vi "Mixed mode s-parameter - change port assignment.vi"(11 "S-parameters in":cdb[][](array[numeric]) format="%#.6g") -> (3 "S-parameters out":cdb[][](array[numeric]) format="%#.6g")   [LabVIEW 2020]
uses:
  <vilib>/addons/HF Network Analysis/Support VIs/Read SnP File (SnP).vi
  <vilib>/addons/HF Network Analysis/NI_HFNetworkAnalysis.lvlib
panel:
  in  "Run Standalone":bool
  in  "SnP File Path":path
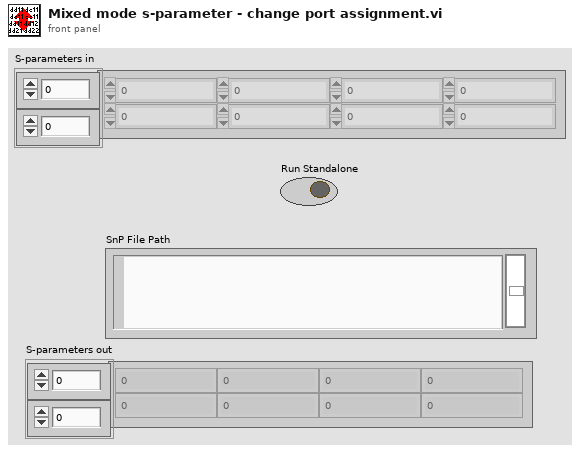
[diagram p1: front panel]
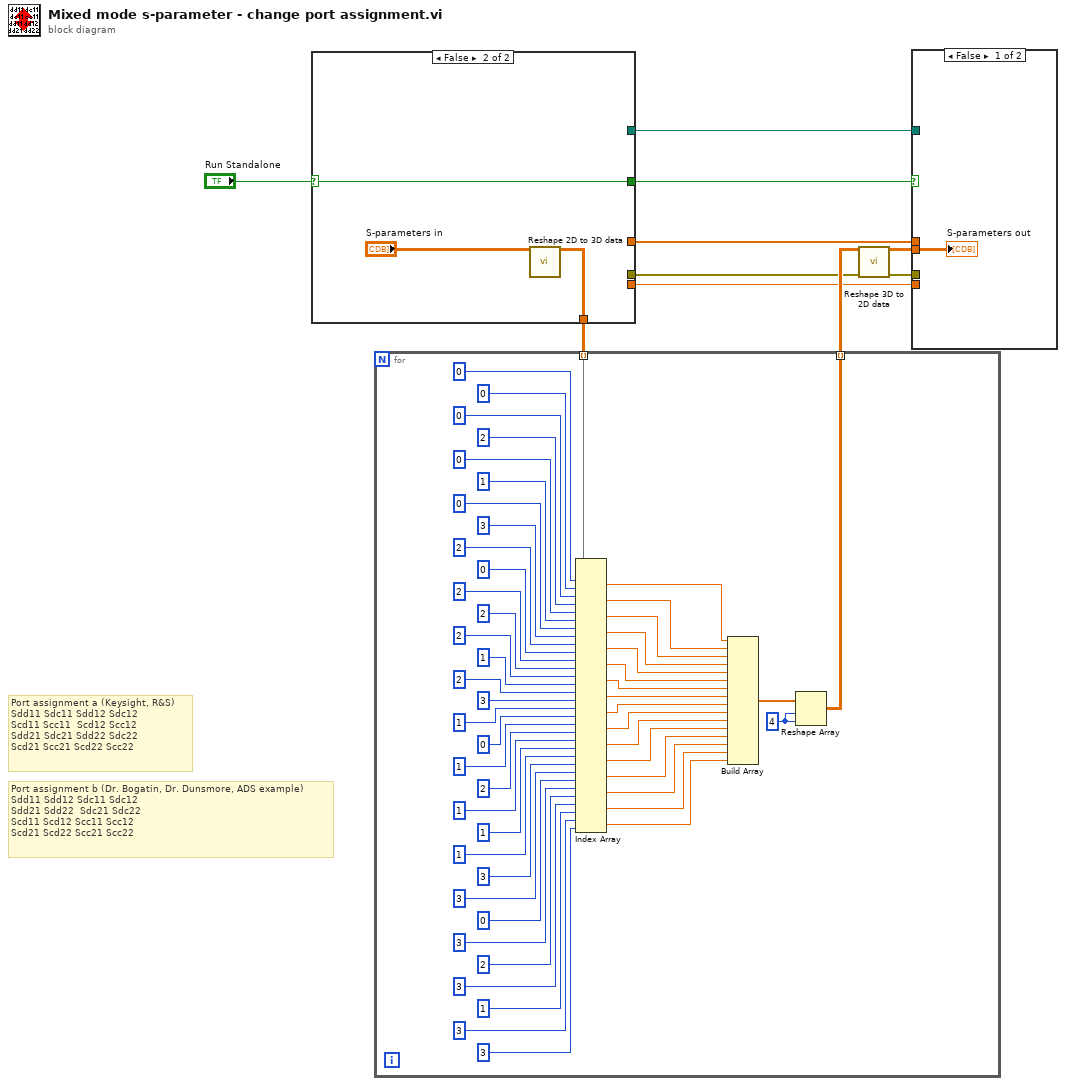
[diagram p0: block diagram]
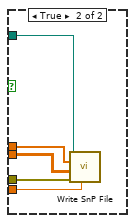
[diagram p2: hidden frame]
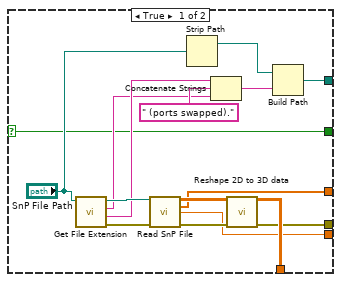
[diagram p3: hidden frame]
diagram:
  # "Port assignment b (Dr. Bogatin, Dr. Dunsmore, ADS example)\nSdd11 Sdd12 Sdc11 Sdc12\nSdd21 Sdd22  Sdc21 Sdc22\nScd11 Scd12 Scc11 Scc12\nScd21 Scd22 Scc21 Scc22"
  # "Port assignment a (Keysight, R&S)\nSdd11 Sdc11 Sdd12 Sdc12\nScd11 Scc11  Scd12 Scc12\nSdd21 Sdc21 Sdd22 Sdc22\nScd21 Scc21 Scd22 Scc22"
  n1 = case shown="False" "Run Standalone" {
    selector: "Run Standalone" -> [w11 w27]
    tunnel: [w22 w29] -> w10
    tunnel: [w15 _] -> w5
    tunnel: [w14 _] -> w4
    tunnel: [w13 _] -> w3
    tunnel: [w12 _] -> w2
    tunnel: [w11 w27] -> w1
    frame True {
      n2 = call <vilib>:"Get File Extension.vi"("file"="SnP File Path") -> ("error out"=w25:errorcluster, "filename without extension"=w21:string, "lowercase file extension"=w19:string, "dup file"=w26:path)  [unwired: 6 in, 1 out]
      n3 = call-poly <vilib>:"Read SnP File.vi"("SnP File Path"=w26, "Error In"=w25) -> ("S-parameters"=w24:cdb[][], "Frequencies (Hz)"=w13:dbl[], "Z0 (Ohm)"=w14:cdb, "Error Out"=w23:errorcluster)  [unwired: 10 in]
      n4 = Strip Path(path="SnP File Path") -> (stripped path=w16:path)  [unwired: 1 out]
      n5 = Concatenate Strings(w21, " (ports swapped)." ("string"), w19) -> (w18:string)
      n6 = call <vilib>:"Reshape 2D to 3D data.vi"("Parameters In (2D)"=w24, "Error In"=w23) -> ("Parameters Out (3D)"=w22:cdb[][][], "Error Out"=w15:errorcluster)  [unwired: 12 in]
      n7 = Build Path(base path=w16, name or relative path=w18) -> (appended path=w12:path)
    }
    frame False {
      n8 = call <vilib>:"Reshape 2D to 3D data.vi"("Parameters In (2D)"="S-parameters in") -> ("Parameters Out (3D)"=w29:cdb[][][])  [unwired: 13 in, 1 out]
    }
  }
  n9 = for {
    tunnel: w10 -> [w31] mode=indexing
    tunnel: [w30] -> w9 mode=indexing
    w64 = 4 ("dimension size")
    n10 = Index Array(array=w31, index (row) #1=0 ("index (row)"), index (col) #1=0 ("disabled index (col)"), index (row) #2=0 ("index (row)"), index (col) #2=2 ("disabled index (col)"), index (row) #3=0 ("index (row)"), index (col) #3=1 ("disabled index (col)"), index (row) #4=0 ("index (row)"), index (col) #4=3 ("disabled index (col)"), index (row) #5=2 ("index (row)"), index (col) #5=0 ("disabled index (col)"), index (row) #6=2 ("index (row)"), index (col) #6=2 ("disabled index (col)"), index (row) #7=2 ("index (row)"), index (col) #7=1 ("disabled index (col)"), index (row) #8=2 ("index (row)"), index (col) #8=3 ("disabled index (col)"), index (row) #9=1 ("index (row)"), index (col) #9=0 ("disabled index (col)"), index (row) #10=1 ("index (row)"), index (col) #10=2 ("disabled index (col)"), index (row) #11=1 ("index (row)"), index (col) #11=1 ("disabled index (col)"), index (row) #12=1 ("index (row)"), index (col) #12=3 ("disabled index (col)"), index (row) #13=3 ("index (row)"), index (col) #13=0 ("disabled index (col)"), index (row) #14=3 ("index (row)"), index (col) #14=2 ("disabled index (col)"), index (row) #15=3 ("index (row)"), index (col) #15=1 ("disabled index (col)"), index (row) #16=3 ("index (row)"), index (col) #16=3 ("disabled index (col)")) -> (element #1=w66:cdb, element #2=w81:cdb, element #3=w80:cdb, element #4=w79:cdb, element #5=w78:cdb, element #6=w77:cdb, element #7=w76:cdb, element #8=w75:cdb, element #9=w74:cdb, element #10=w73:cdb, element #11=w72:cdb, element #12=w71:cdb, element #13=w67:cdb, element #14=w70:cdb, element #15=w69:cdb, element #16=w68:cdb)
    n11 = Build Array(w66, w81, w80, w79, w78, w77, w76, w75, w74, w73, w72, w71, w67, w70, w69, w68) -> (w65:cdb[])
    n12 = Reshape Array(w65, w64, w64) -> (w30:cdb[][])
  }
  n13 = call <vilib>:"Reshape 3D to 2D data.vi"("Parameters In (3D)"=w9, "Error In"=w5) -> ("Parameters Out (2D)"=w6:cdb[][], "Error Out"=w7:errorcluster)  [unwired: 12 in]
  n14 = case shown="False" w1 {
    tunnel: w7 -> [_ w87]
    tunnel: w6 -> [w82 w86]
    tunnel: w4 -> [_ w85]
    tunnel: w3 -> [_ w84]
    tunnel: w2 -> [_ w83]
    frame False {
      "S-parameters out" <- w82
    }
    frame True {
      n15 = call <vilib>:"Write SnP File.vi"("Z0 (50 Ohm)"=w85, "error in (no error)"=w87, "S-parameters"=w86, "Frequencies (Hz)"=w84, "SnP File Path"=w83) -> ()  [unwired: 6 in, 1 out]
    }
  }
